vi "CheckSHOT_atSHIP.vi"(8 "ShipRectangle":T1, 11 "InvaderShotArray":T2(array[cluster])) -> (3 "SHOT":bool)   [LabVIEW 2019]
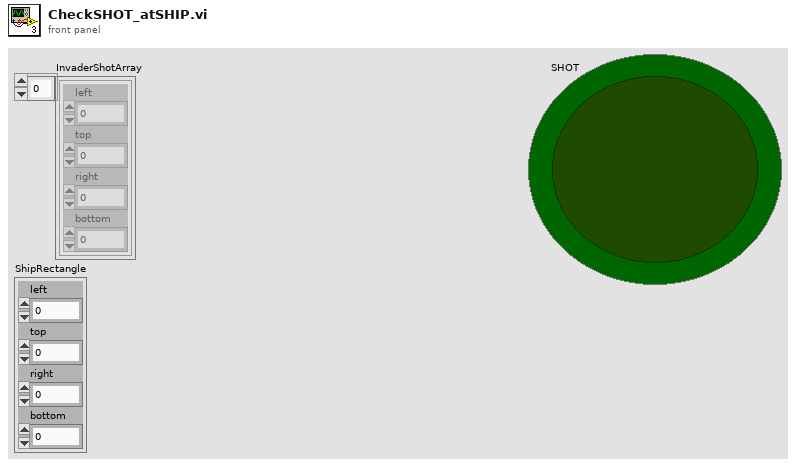
[diagram p1: front panel]
types:
  T1 = cluster{"left":i16, "top":i16, "right":i16, "bottom":i16}
  T2 = cluster{"left":i16, "top":i16, "right":i16, "bottom":i16}[]
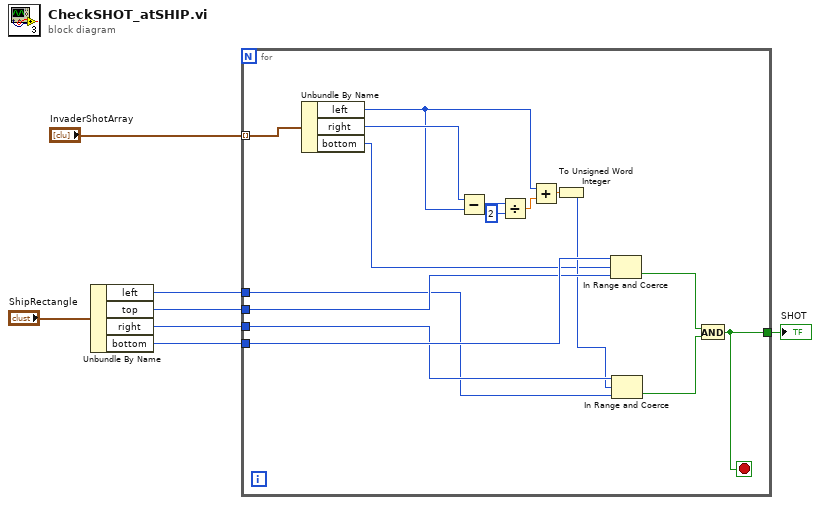
[diagram p0: block diagram]
diagram:
  n1 = Unbundle By Name("ShipRectangle") -> ("left"=w2:i16, "top"=w6:i16, "right"=w3:i16, "bottom"=w5:i16)
  n2 = for {
    tunnel: "InvaderShotArray" -> [w23] mode=indexing
    tunnel: w2 -> [w16]
    tunnel: w6 -> [w21]
    tunnel: w3 -> [w20]
    tunnel: w5 -> [w22]
    tunnel: [w17] -> w4
    stop <- w17 stop-if-true
    n3 = Unbundle By Name(w23) -> ("left"=w10:i16, "right"=w11:i16, "bottom"=w8:i16)
    n4 = Subtract(x=w11, y=w10) -> (x-y=w13:i16)
    n5 = Divide(x=w13, y=i16 2) -> (x/y=w14:dbl)
    n6 = Add(x=w10, y=w14) -> (x+y=w15:dbl)
    n7 = To Unsigned Word Integer(number=w15) -> (unsigned 16bit integer=w9:u16)
    n8 = In Range and Coerce(upper limit=w22, x=w8, lower limit=w21) -> (In Range?=w19:bool)  [unwired: 1 out]
    n9 = In Range and Coerce(upper limit=w20, x=w9, lower limit=w16) -> (In Range?=w18:bool)  [unwired: 1 out]
    n10 = And(x=w19, y=w18) -> (x .and. y?=w17:bool)
  }
  "SHOT" <- w4
